vi "Stop Application.vi"(11 "error in (no error)":errorcluster) -> (15 "error out":errorcluster)   [LabVIEW 2014, in "Coding Platform.lvlib"]
uses:
  Coding Platform.lvlib
  Typedefs/User Event Operations.ctl
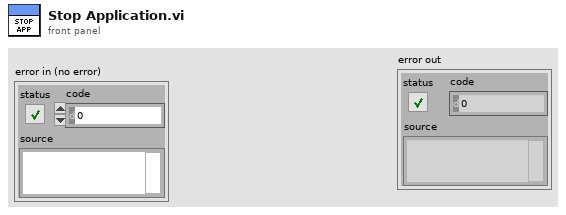
[diagram p1: front panel]
types:
  T1 = typedef "Coding Platform.lvlib/User Event Operations.ctl" = enum16{"Create", "Genereate", "Destroy", "Get Reference"}
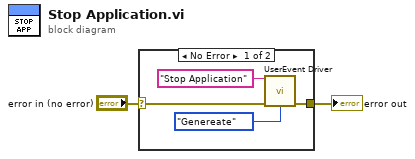
[diagram p0: block diagram]
diagram:
  n1 = case shown="No Error" "error in (no error)" {
    selector: "error in (no error)" -> [w3 w7]
    tunnel: [w6 w7] -> w2
    frame No Error {
      n2 = call "UserEvent Driver.vi"("Message"="Stop Application", "error in (no error)"=w3, "Operations(Get Reference)"=User_Event_Operations."Genereate") -> ("error out"=w6:errorcluster)  [unwired: 11 in, 1 out]
    }
    frame Error {
    }
  }
  "error out" <- w2
